vi "EXPERIMENTAL_CAPTURE_LATCHING.vi"() -> ()   [LabVIEW 2019]
uses:
  <vilib>/numeric/Random Number (Range) DBL.vi
  <vilib>/Utility/file.llb/Write Delimited Spreadsheet (string).vi
panel:
  in  "stop":bool
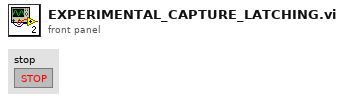
[diagram p1: front panel]
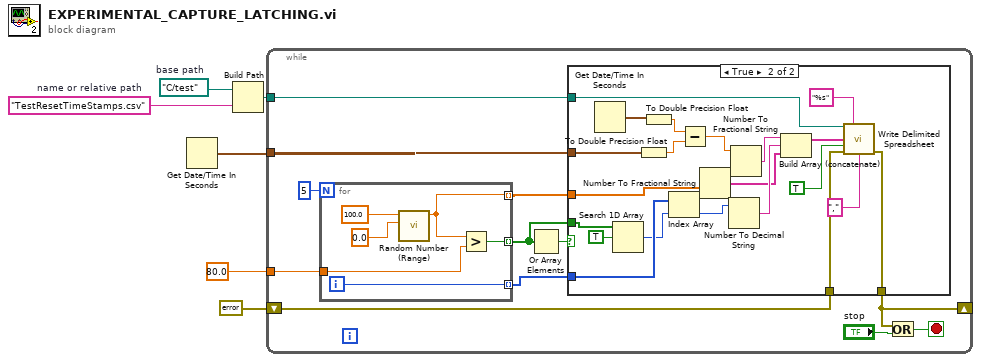
[diagram p0: block diagram]
diagram:
  w4 = "TestResetTimeStamps.csv"  # name or relative path
  w5 = path "C:/test"  # base path
  n1 = Get Date/Time In Seconds() -> (seconds since 1Jan1904=w2:timestamp)
  n2 = Build Path(base path=w5, name or relative path=w4) -> (appended path=w6:path)
  n3 = while {
    tunnel: w6 -> [w18]
    shift-right: [w15] -> _
    shift-left: errorcluster {"status"=FALSE, "code"=0, "source"=""} ("error in (no error)") -> [w17]
    tunnel: w2 -> [w16]
    tunnel: 80.0 -> [w12]
    stop <- w13 stop-if-true
    n4 = for {
      N: 5 -> [_]
      tunnel: [w24] -> w9 mode=indexing
      tunnel: w12 -> [w21]
      tunnel: [w20] -> w8 mode=indexing
      tunnel: [w19] -> w7 mode=indexing
      i -> [w20]
      n5 = call-poly <vilib>:"Random Number (Range).vi"("lower bound (0)"=0.0 ("0"), "upper bound (100)"=100.0) -> ("number"=w19:dbl)  [unwired: 9 in]
      n6 = Greater?(x=w19, y=w21) -> (0:w24:bool)
    }
    n7 = Or Array Elements(Boolean array=w9) -> (logical OR=w10:bool)
    n8 = case shown="True" w10 {
      tunnel: w18 -> [_ w46]
      tunnel: w17 -> [w25 w45]
      tunnel: [w25 w44] -> w15
      tunnel: w16 -> [_ w39]
      tunnel: w9 -> [_ w36]
      tunnel: w8 -> [_ w34]
      tunnel: w7 -> [_ w27]
      frame False {
      }
      frame True {
        n9 = Get Date/Time In Seconds() -> (seconds since 1Jan1904=w40:timestamp)
        n10 = Search 1D Array(1D array=w36, element=TRUE) -> (index of element=w33:i32)  [unwired: 1 in]
        n11 = To Double Precision Float(number=w39) -> (double precision float=w41:dbl)
        n12 = To Double Precision Float(number=w40) -> (double precision float=w42:dbl)
        n13 = Index Array(array=w34, index=w33) -> (element=w31:i32)
        n14 = Subtract(x=w42, y=w41) -> (x-y=w32:dbl)
        n15 = Number To Fractional String(number=w27) -> (F-format string=w26:string[])  [unwired: 3 in]
        n16 = Number To Decimal String(number=w31) -> (decimal integer string=w29:string)  [unwired: 1 in]
        n17 = Number To Fractional String(number=w32) -> (F-format string=w30:string)  [unwired: 3 in]
        n18 = Build Array (concatenate)(w30, w29, w26) -> (w38:string[])
        n19 = call-poly <vilib>:"Write Delimited Spreadsheet.vi"("file path (dialog if empty)"=w46, "format (%s)"="%s" ("format (%.3f)"), "1D data"=w38, "append to file? (new file:F)"=TRUE, "error in (no error)"=w45, "delimiter (\\t)"="," ("delimiter (\\t)")) -> ("error out"=w44:errorcluster)  [unwired: 8 in, 1 out]
      }
    }
    n20 = Or(x=w15, y="stop") -> (x .or. y?=w13:bool)
  }
